vi "svfa_Check for Window Change.vi"(6 "window":T1 items=["None"=0, "Hanning"=1, "Hamming"=2, "Blackman-Harris"=3, "Exact Blackman"=4, "Blackman"=5, "Flat Top"=6, "4 Term B-Harris "=7, "7 Term B-Harris"=8, "Low Sidelobe"=9, "Force"=64, "Exponential"=65, "Blackman Nuttall"=11, "Triangle"=30, "Bartlett-Hanning"=31, "Bohman"=32, "Parzen"=33, "Welch"=34, "Kaiser"=60, "Dolph-Chebyshev"=61, "Gaussian"=62], 7 "restart averaging (F)":bool, 8 "error in (no error)":errorcluster) -> (0 "error out":errorcluster, 2 "parameter has changed":bool)   [LabVIEW 2017]
uses:
  <vilib>/addons/_NISVFA/_Shared subVIs/Controls/svc_Window.ctl
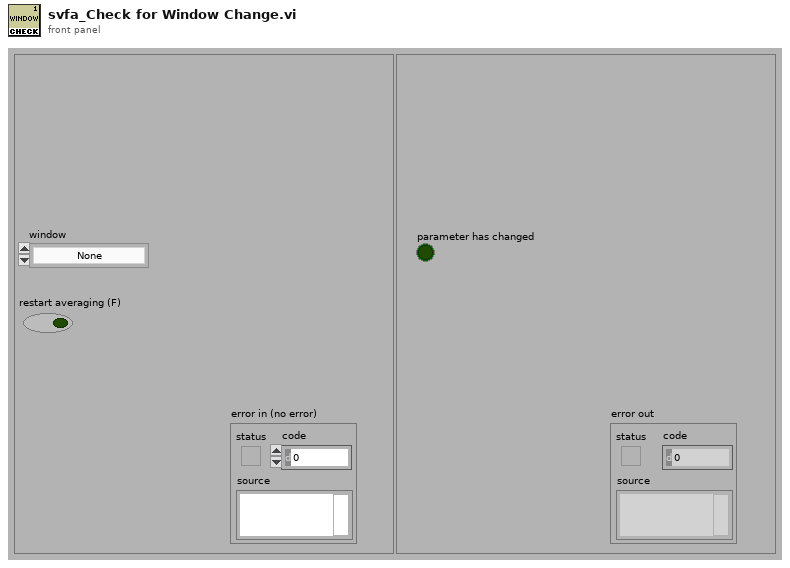
[diagram p1: front panel]
types:
  T1 = typedef "svc_Window.ctl" = u32
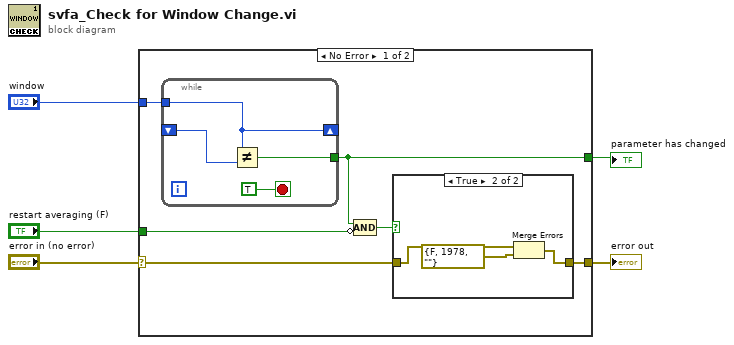
[diagram p0: block diagram]
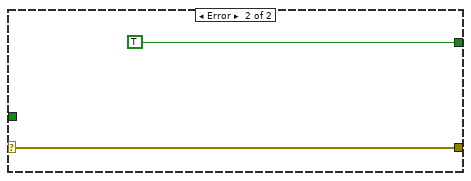
[diagram p3: hidden frame]
diagram:
  n1 = case shown="No Error" "error in (no error)" {
    selector: "error in (no error)" -> [w10 w21]
    tunnel: [w9 w21] -> w4
    tunnel: "window" -> [w11 _]
    tunnel: [w6 TRUE] -> w2
    tunnel: "restart averaging (F)" -> [w8 _]
    frame No Error {
      n2 = while {
        tunnel: w11 -> [w12]
        tunnel: [w14] -> w6
        shift-left: _ -> [w13]
        shift-right: [w12] -> _
        stop <- TRUE stop-if-true
        n3 = Not Equal?(x=w12, y=w13) -> (x != y?=w14:bool)
      }
      n4 = Compound Arithmetic op=AND(w6, invert w8) -> (w7:bool)
      n5 = case shown="True" w7 {
        tunnel: w10 -> [w16 w19]
        tunnel: [w16 w17] -> w9
        frame False {
        }
        frame True {
          n6 = Merge Errors(w19, errorcluster {"status"=FALSE, "code"=1978, "source"=""} ("error IO")) -> (w17:errorcluster)
        }
      }
    }
    frame Error {
    }
  }
  "error out" <- w4
  "parameter has changed" <- w2
